vi "Load Ungoaled Categories.vi"(8 "error in (no error)":errorcluster, 10 "Year-Mo":string, 11 "Database in":refnum<class "Database.lvclass">) -> (0 "error out":errorcluster, 2 "Categories with No Goal":refnum<class "Category.lvclass">[](array[class]), 3 "Database out":refnum<class "Database.lvclass">)   [LabVIEW 2018, in "Database.lvclass"]
uses:
  Database.lvclass
  Category/Category.lvclass
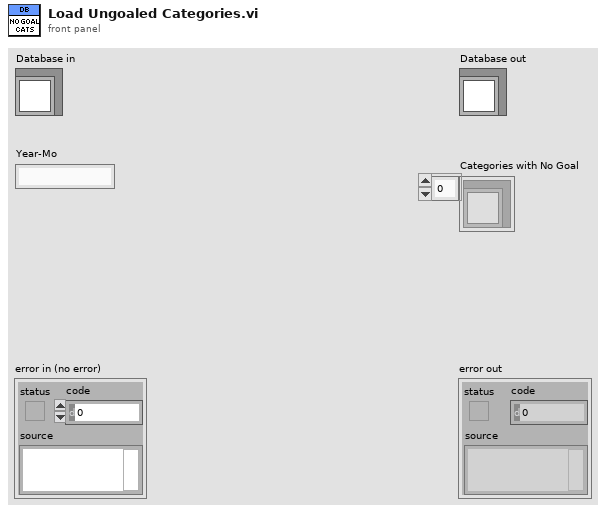
[diagram p1: front panel]
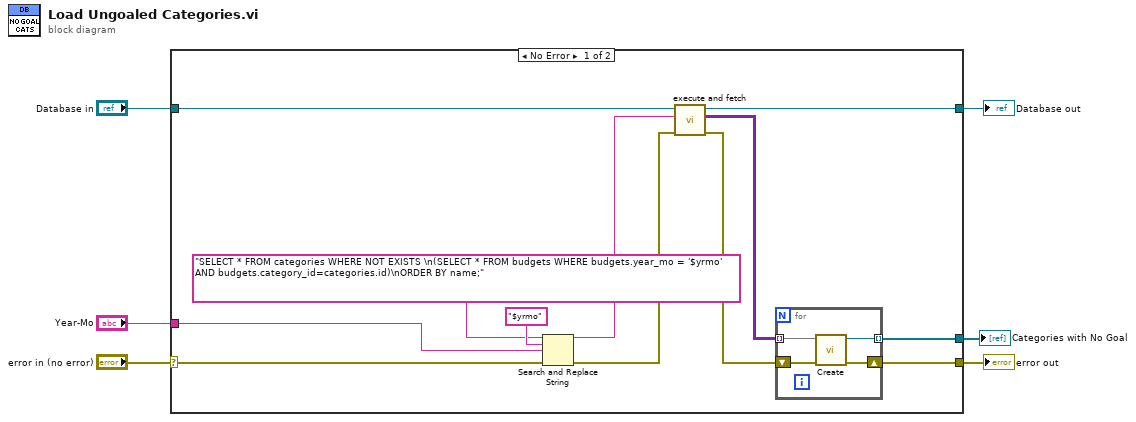
[diagram p0: block diagram]
diagram:
  n1 = case shown="No Error" "error in (no error)" {
    selector: "error in (no error)" -> [w17 w24]
    tunnel: [w11 w24] -> w5
    tunnel: [w12 w23] -> w3
    tunnel: "Database in" -> [w9 w23]
    tunnel: [w10 _] -> w2
    tunnel: "Year-Mo" -> [w7 _]
    frame No Error {
      n2 = Search and Replace String(input string="SELECT * FROM categories WHERE NOT EXISTS \n(SELECT * FROM budgets WHERE budgets.year_mo = '$yrmo' AND budgets.category_id=categories.id)\nORDER BY name;", search string="$yrmo", replace string=w7, error in=w17) -> (result string=w13:string, error out=w14:errorcluster)  [unwired: 4 in, 2 out]
      n3 = call "execute and fetch.vi"("error in (no error)"=w14, "SQL query"=w13, "Database in"=w9) -> ("error out"=w15:errorcluster, "recordset data"=w16:variant[][], "Database out"=w12:refnum<class "Database.lvclass">)  [unwired: 5 in, 1 out]
      n4 = for {
        tunnel: w16 -> [w22] mode=indexing
        shift-right: [w19] -> w11
        shift-left: w15 -> [w21]
        tunnel: [w20] -> w10 mode=indexing
        n5 = call "Create.vi"("error in (no error)"=w21, "Record"=w22) -> ("error out"=w19:errorcluster, "Category out"=w20:refnum<class "Category.lvclass">)  [unwired: 8 in]
      }
    }
    frame Error {
    }
  }
  "error out" <- w5
  "Database out" <- w3
  "Categories with No Goal" <- w2
